vi "store catch block.vi"(8 "error in":errorcluster, 10 "reg":enum16{"reg 1", "reg 2", "reg 3"}(ring), 11 "store/catch":enum16{"store", "catch out"}(ring)) -> (0 "error out":errorcluster)   [LabVIEW 2019]
uses:
  ctl/servo act.ctl
  ctl/height.ctl
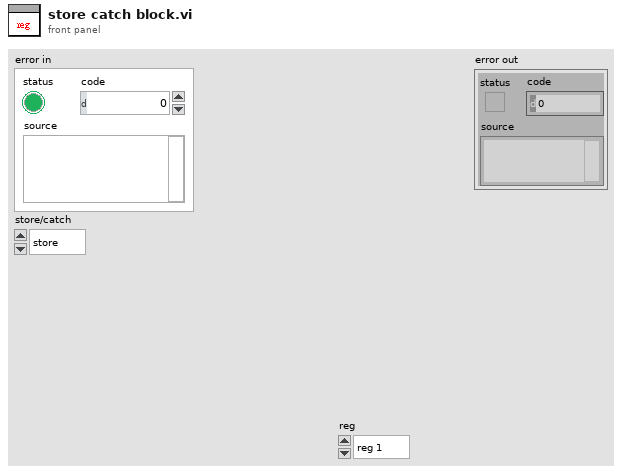
[diagram p1: front panel]
types:
  T1 = typedef "servo act.ctl" = enum16{"catch", "relax", "left idle", "center", "red relax", "left reg", "right reg"}
  T2 = typedef "height.ctl" = enum16{"IDLE", "recycle pre-catch", "recycle catch", "recycle zone", "vision height", "box 1", "box 2", "box 3", "box 1 pre", "box 2 pre", "box 3 pre", "reg 1", "reg 2", "reg 1 pre", "reg 2 pre", "put 1", "put 2", "put 3"}
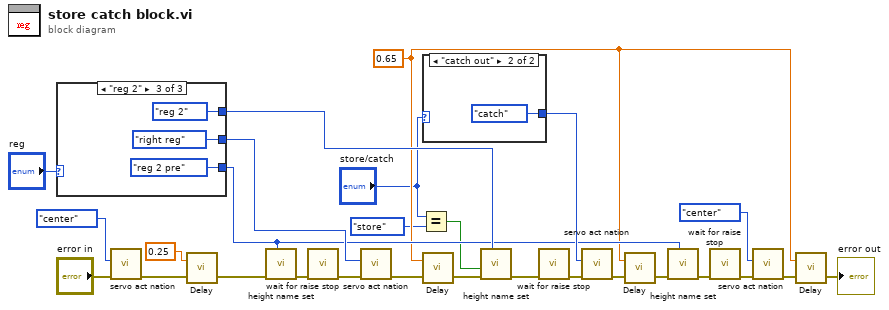
[diagram p0: block diagram]
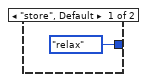
[diagram p2: hidden frame]
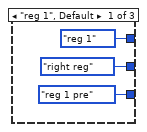
[diagram p3: hidden frame]
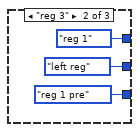
[diagram p4: hidden frame]
diagram:
  w6 = 0.65 ("Delay Time (s)")
  n1 = case shown="\"reg 2\"" "reg" {
    tunnel: [height."reg 1 pre" ("height name") height."reg 1 pre" ("height name") height."reg 2 pre" ("height name")] -> w11
    tunnel: [servo_act."right reg" ("servo act") servo_act."left reg" ("servo act") servo_act."right reg" ("servo act")] -> w19
    tunnel: [height."reg 1" ("height name") height."reg 1" ("height name") height."reg 2" ("height name")] -> w18
    frame "reg 1", Default {
    }
    frame "reg 3" {
    }
    frame "reg 2" {
    }
  }
  n2 = call "servo act nation.vi"("error in"="error in", "servo act"=servo_act."center") -> ("error out"=w25:errorcluster)  [unwired: 9 in]
  n3 = call "Delay.vi"("error in (no error)"=w25, "Delay Time (s)"=0.25) -> ("error out"=w23:errorcluster)  [unwired: 1 in]
  n4 = call "height name set.vi"("height name"=w11, "error in (no error)"=w23) -> ("error out"=w21:errorcluster)  [unwired: 9 in]
  n5 = call "wait for raise stop.vi"("Error In"=w21) -> ("Error Out"=w20:errorcluster)  [unwired: 10 in]
  n6 = call "servo act nation.vi"("error in"=w20, "servo act"=w19) -> ("error out"=w16:errorcluster)  [unwired: 9 in]
  n7 = Equal?(x="store/catch", y=enum16{"store", "catch out"}."store") -> (x = y?=w1:bool)
  n8 = case shown="\"catch out\"" "store/catch" {
    tunnel: [servo_act."relax" ("servo act") servo_act."catch" ("servo act")] -> w14
    frame "store", Default {
    }
    frame "catch out" {
    }
  }
  n9 = call "Delay.vi"("error in (no error)"=w16, "Delay Time (s)"=w6) -> ("error out"=w17:errorcluster)  [unwired: 1 in]
  n10 = call "height name set.vi"("height name"=w18, "error in (no error)"=w17, "plus 2"=w1) -> ("error out"=w2:errorcluster)  [unwired: 8 in]
  n11 = call "wait for raise stop.vi"("Error In"=w2) -> ("Error Out"=w15:errorcluster)  [unwired: 10 in]
  n12 = call "servo act nation.vi"("error in"=w15, "servo act"=w14) -> ("error out"=w13:errorcluster)  [unwired: 9 in]
  n13 = call "Delay.vi"("error in (no error)"=w13, "Delay Time (s)"=w6) -> ("error out"=w12:errorcluster)  [unwired: 1 in]
  n14 = call "height name set.vi"("height name"=w11, "error in (no error)"=w12) -> ("error out"=w10:errorcluster)  [unwired: 9 in]
  n15 = call "wait for raise stop.vi"("Error In"=w10) -> ("Error Out"=w9:errorcluster)  [unwired: 10 in]
  n16 = call "servo act nation.vi"("error in"=w9, "servo act"=servo_act."center") -> ("error out"=w7:errorcluster)  [unwired: 9 in]
  n17 = call "Delay.vi"("error in (no error)"=w7, "Delay Time (s)"=w6) -> ("error out"=→"error out":errorcluster)  [unwired: 1 in]
